vi "GUI_Plasma2SuperGUI.vi"() -> ()   [LabVIEW 2011]
uses:
  GUI_Template/GUI_master/tcp_new_data_event.ctl
  GUI_Template/GUI_master/tcp new data cluster.ctl
  Device Driver/DG645/subVIs/TriggerSource_TypDef.ctl
  <vilib>/vision/NI_Vision_Development_Module.lvlib
panel:
  in  "Tab Control":enum32{"ref", "BG subtracted"}(tab)
  out "background image":T1(plugin-control)
  out "Image":T1(plugin-control)
  out "error out":errorcluster
  in  "make ref":bool
  in  "trigger::1":bool caption="Trigger"
  in  "Disable AASC Valve Trigger":bool caption="Disable Valve Trigger"
  in  "Trigger Control":enum32{"Trigger", "Single Shot"}(tab)
  in  "Trigger.Rate::2":dbl=0.001 caption="Trigger Rate [Hz]" min=0.001 max=1000.0 format="%_2f"
  in  "Fire":bool
  in  "fire::2":string caption="Fire Status"
  in  "Trigger.Source::2":T2 caption="Trigger Source"
  in  "Delay.Ch C::2":dbl=0.001 caption="Valve Trigger Timing [s] Ch_CD" min=-0.1 max=0.1 format="%.9f"
  in  "Delay.Ch A::2":dbl=0.001 caption="Phasics Trigger Timing [s] Ch_AB" min=-0.1 max=0.1 format="%.9f"
  in  "Trigger.Level::2":dbl=0.001 caption="Trigger Level" min=0.5 max=4.0 format="%_4f"
  in  "uangle::3":dbl=0.001 caption="u angle [deg]" min=-1.0 max=1.0 format="%_4p"
  in  "vangle::3":dbl=0.001 caption="v angle [deg]" min=-1.0 max=1.0 format="%_4p"
  in  "wangle::3":dbl=0.001 caption="w angle [deg]" min=-1.0 max=1.0 format="%_4p"
  in  "ypos::3":dbl=0.001 caption="hex y [mm]" min=-15.0 max=15.0 format="%_4p"
  in  "zpos::3":dbl=0.001 caption="hex z [mm]" min=-12.0 max=12.0 format="%_4p"
  in  "xpos::3":dbl=0.001 caption="hex x [mm]" min=-15.0 max=15.0 format="%_4p"
  in  "parameter::4":string caption="Jet Backing Pressure [PSIG]"
  in  "GUIdevice 4":string="P2-HP-pressure"
  in  "GUIdevice 3":string="P2_hexapod"
  in  "Amplitude.Ch CD::2":dbl=0.001 caption="Ch CD Amplitude" min=0.5 max=5.0 format="%_4f"
  in  "Amplitude.Ch AB::2":dbl=0.001 caption="Ch AB Amplitude" min=0.5 max=5.0 format="%_4f"
  in  "GUIdevice 2":string="P2_DDG"
  in  "stop":bool
  in  "gain::1":dbl=0.001 caption="gain" min=40.0 max=210.0 format="%_4f"
  in  "exposure::1":dbl=0.001 caption="exposure" min=0.0 max=7.0 format="%_4p"
  out "image::1":T1(plugin-control) caption="Phasics Cam"
  in  "GUIdevice 1":string="P2-phasics"
  out "tcp data event":T3
  out "error IO 2":errorcluster
  # "Timing Box Control"
  # "Hexapod Control"
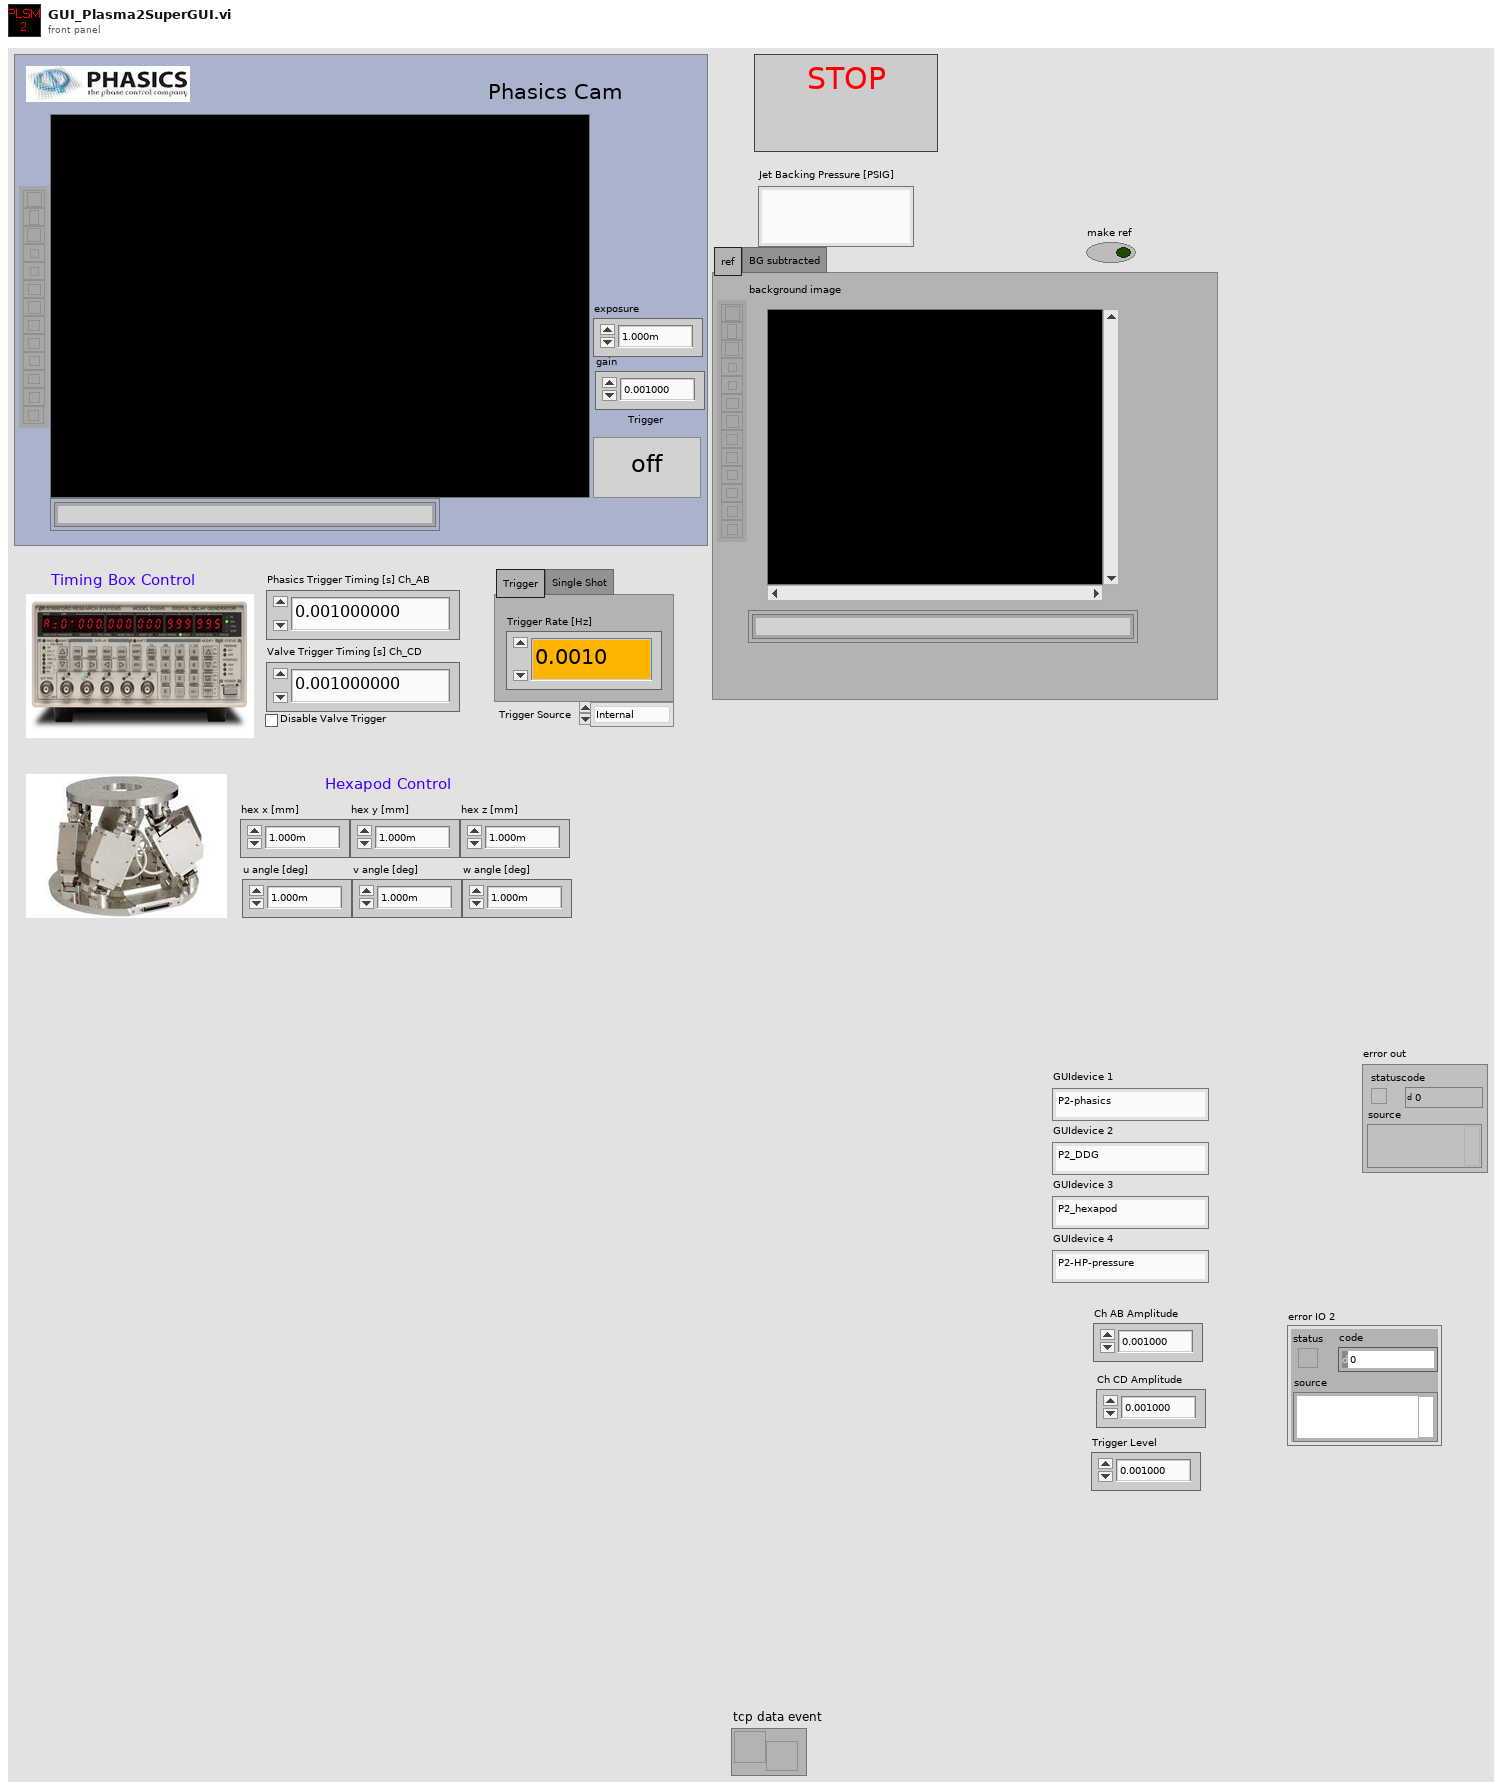
[diagram p1: front panel]
types:
  T1 = typedef "IMAQ Image.ctl" = refnum<image>
  T2 = typedef "TriggerSource_TypDef.ctl" = enum16{"Internal", "External rising edges", "External falling edges", "Single shot external rising edges", "Single shot external falling edges", "Single shot", "Line"}
  T3 = typedef "tcp_new_data_event.ctl" = refnum<user-event>
  T4 = typedef "Image Type" = u32
  T5 = typedef "tcp new data cluster.ctl" = cluster{"EventEnum":enum16{"new data", "connection status update"}, "Device name":string}
  T6 = enum16{"Internal", "External rising edges", "External falling edges", "Single shot external rising edges", "Single shot external falling edges", "Single shot", "Line"}
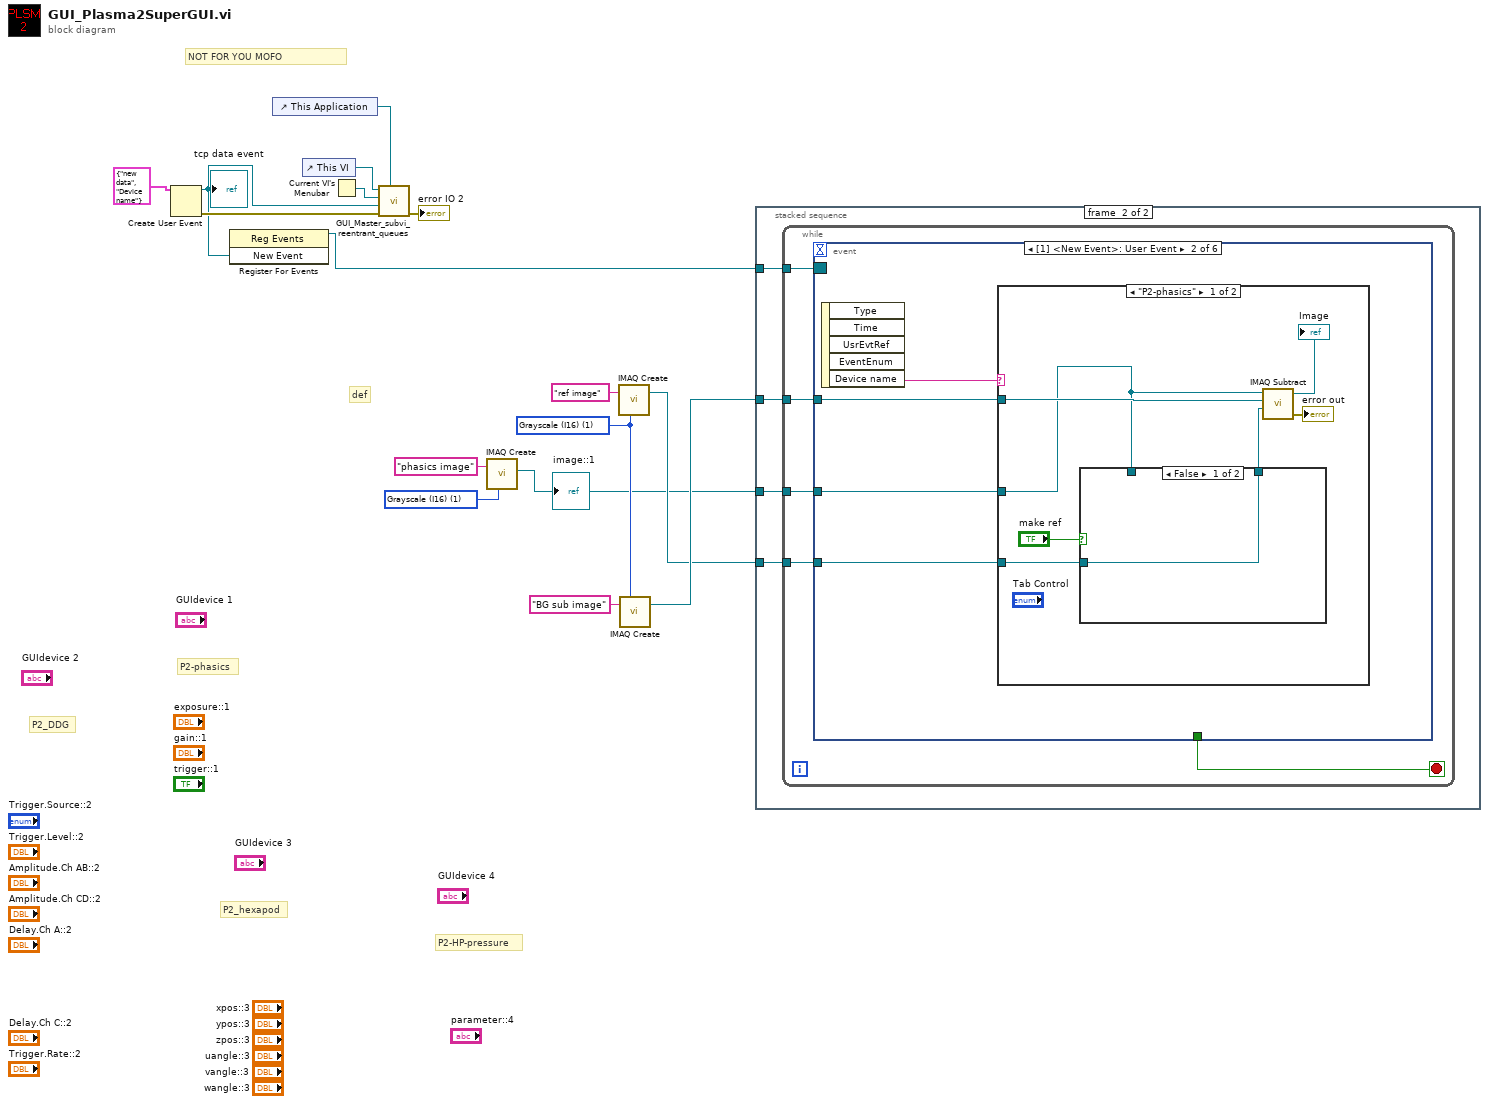
[diagram p0: block diagram]
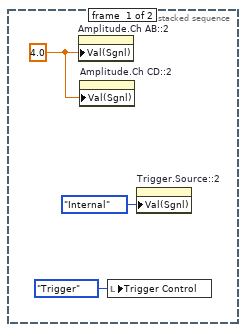
[diagram p2: hidden frame]
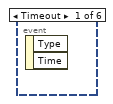
[diagram p3: hidden frame]
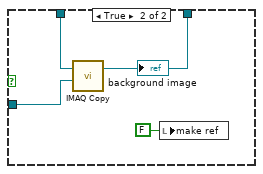
[diagram p4: hidden frame]
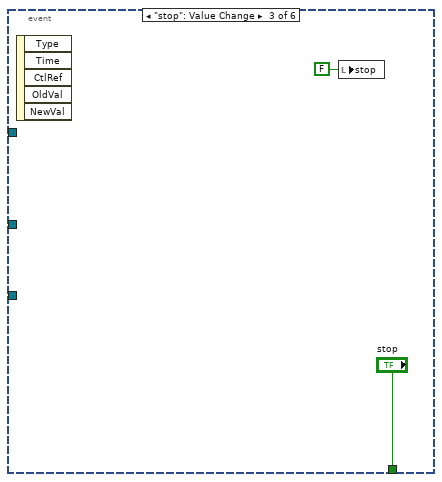
[diagram p6: hidden frame]
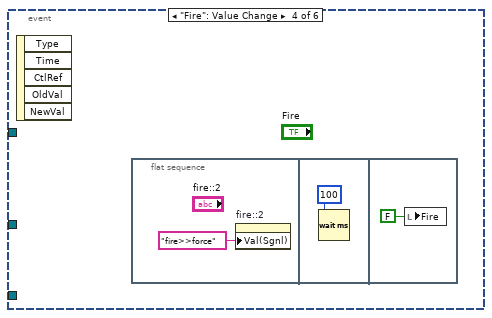
[diagram p7: hidden frame]
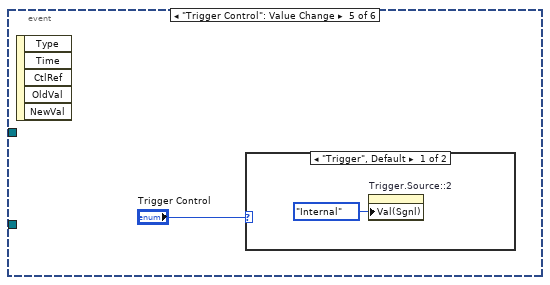
[diagram p8: hidden frame]
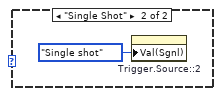
[diagram p9: hidden frame]
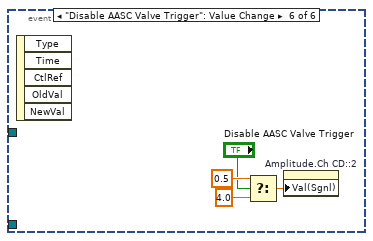
[diagram p10: hidden frame]
diagram:
  w3 = T4 1 items=["Grayscale (U8)", "Grayscale (I16)", "Grayscale (SGL)", "Complex (CSG)", "RGB (U32)", "HSL (U32)", "RGB (U64)", "Grayscale (U16)"] ("Image Type")
  w5 = T4 1 items=["Grayscale (U8)", "Grayscale (I16)", "Grayscale (SGL)", "Complex (CSG)", "RGB (U32)", "HSL (U32)", "RGB (U64)", "Grayscale (U16)"] ("Image Type")
  # "def"
  # "P2-phasics"
  # "P2-HP-pressure"
  # "P2_hexapod"
  # "P2_DDG"
  # "NOT FOR YOU MOFO"
  n1 = Create User Event(user event datatype=T5 {"EventEnum"=enum."new data", "Device name"="Device name"} ("New Event")) -> (user event=w11:refnum<user-event>, error out=w12:errorcluster)  [unwired: 1 in]
  "tcp data event" <- w11
  n2 = register-events(w11) -> (reference out=w9:refnum<event-registration>)  [unwired: 2 in, 1 out]
  n3 = control-ref of="This Application"() -> (w10:refnum<vi>)
  n4 = control-ref of="This VI"() -> (w15:refnum<vi>)
  n5 = Current VI's Menubar() -> (w14:refnum<k9>)
  n6 = call "GUI_Master_subvi_reentrant_queues.vi"("This Application"=w10, "error in (no error)"=w12, "tcp data event"=w11, "Caller menu reference"=w14, "Caller VI ref"=w15) -> ("error out"=→"error IO 2":errorcluster)  [unwired: 6 in]
  n7 = call "IMAQ Create"("Image Name"="phasics image", "Image Type"=w3) -> ("New Image"=w1:T1)  [unwired: 3 in, 1 out]
  "image::1" <- w1
  n8 = call "IMAQ Create"("Image Name"="ref image", "Image Type"=w5) -> ("New Image"=w4:T1)  [unwired: 3 in, 1 out]
  n9 = call "IMAQ Create"("Image Name"="BG sub image", "Image Type"=w5) -> ("New Image"=w6:T1)  [unwired: 3 in, 1 out]
  n10 = stacked-sequence {
    tunnel: w9 -> [_ w23]
    tunnel: w6 -> [_ w22]
    tunnel: w4 -> [_ w21]
    tunnel: w1 -> [_ w20]
    frame #0 {
      w18 = 4.0 ("Value (Signaling)")
      n11 = property on="Amplitude.Ch AB::2" class="DigNum (strict)"("Val(Sgnl)"=w18) -> ()  [unwired: 2 in, 2 out]
      n12 = property on="Amplitude.Ch CD::2" class="DigNum (strict)"("Val(Sgnl)"=w18) -> ()  [unwired: 2 in, 2 out]
      n13 = local write "Trigger Control"(enum32{"Trigger", "Single Shot"}."Trigger" ("Trigger Control")) -> ()
      n14 = property on="Trigger.Source::2" class="Enum (strict)"("Val(Sgnl)"=T6."Internal" ("Value (Signaling)")) -> ()  [unwired: 2 in, 2 out]
    }
    frame #1 {
      n15 = while {
        tunnel: w23 -> [w27]
        tunnel: w22 -> [w26]
        tunnel: w21 -> [w25]
        tunnel: w20 -> [w24]
        stop <- w28 stop-if-true
        n16 = event shown="[1] <New Event>: User Event" {
          selector: w27 -> [_ _ _ _ _ _]
          dyn-events: _ -> [_ _ _ _ _ _]
          timeout: _ -> [_ _ _ _ _ _]
          tunnel: [_ _ "stop" _ _ _] -> w28
          tunnel: w26 -> [_ w31 _ _ _ _]
          tunnel: w25 -> [_ w30 _ _ _ _]
          tunnel: w24 -> [_ w29 _ _ _ _]
          event Timeout {
            n17 = event-data() -> ()  [unwired: 1 in, 2 out]
          }
          event User Event {
            n18 = event-data() -> ("Device name"=w32:string)  [unwired: 1 in, 4 out]
            n19 = case shown="\"P2-phasics\"" w32 {
              tunnel: w31 -> [w37 _]
              tunnel: w30 -> [w35 _]
              tunnel: w29 -> [w33 _]
              frame "P2-phasics" {
                n20 = case shown="False" "make ref" {
                  tunnel: w33 -> [_ w44]
                  tunnel: [w40 w42] -> w38
                  tunnel: w35 -> [w40 w43]
                  frame False {
                  }
                  frame True {
                    n21 = call "IMAQ Copy"("Image Dst"=w43, "Image Src"=w44) -> ("Image Dst Out"=w42:T1)  [unwired: 4 in, 1 out]
                    "background image" <- w42
                    n22 = local write "make ref"(FALSE ("make ref")) -> ()
                  }
                }
                n23 = call "IMAQ Subtract"("Image Src A"=w33, "Image Dst"=w37, "Image Src B"=w38) -> ("Image Dst Out"=→"Image":T1, "error out"=→"error out":errorcluster)  [unwired: 4 in]
              }
              frame Default {
              }
            }
          }
          event "stop": Value Change {
            n24 = event-data() -> ()  [unwired: 1 in, 5 out]
            n25 = local write "stop"(FALSE ("stop")) -> ()
          }
          event "Fire": Value Change {
            n26 = event-data() -> ()  [unwired: 1 in, 5 out]
            n27 = flat-sequence {
              frame #0 {
                n28 = property on="fire::2" class="Str"("Val(Sgnl)"="fire>>force" ("Value (Signaling)")) -> ()  [unwired: 2 in, 2 out]
              }
              frame #1 {
                n29 = Wait (ms)(milliseconds to wait=u32 100) -> ()  [unwired: 1 out]
              }
              frame #2 {
                n30 = local write "Fire"(FALSE ("Fire")) -> ()
              }
            }
          }
          event "Trigger Control": Value Change {
            n31 = event-data() -> ()  [unwired: 1 in, 5 out]
            n32 = case shown="\"Trigger\", Default" "Trigger Control" {
              frame "Trigger", Default {
                n33 = property on="Trigger.Source::2" class="Enum (strict)"("Val(Sgnl)"=T6."Internal" ("Value (Signaling)")) -> ()  [unwired: 2 in, 2 out]
              }
              frame "Single Shot" {
                n34 = property on="Trigger.Source::2" class="Enum (strict)"("Val(Sgnl)"=T6."Single shot" ("Value (Signaling)")) -> ()  [unwired: 2 in, 2 out]
              }
            }
          }
          event "Disable AASC Valve Trigger": Value Change {
            n35 = event-data() -> ()  [unwired: 1 in, 5 out]
            n36 = Select(t=0.5 ("Value (Signaling)"), s="Disable AASC Valve Trigger", f=4.0) -> (s? t:f=w56:dbl)
            n37 = property on="Amplitude.Ch CD::2" class="DigNum (strict)"("Val(Sgnl)"=w56) -> ()  [unwired: 2 in, 2 out]
          }
        }
      }
    }
  }
